vi "strip zeroes.vi"(1 "Array in":dbl[](array[numeric])) -> (0 "Array out":dbl[](array[numeric]))   [LabVIEW 2009]
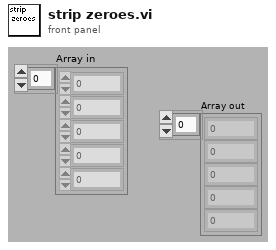
[diagram p1: front panel]
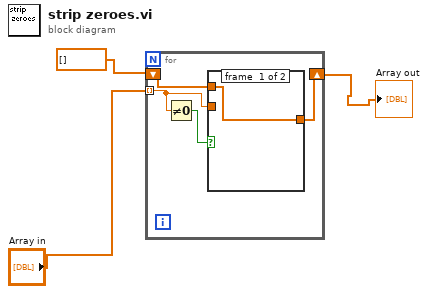
[diagram p0: block diagram]
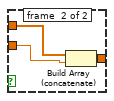
[diagram p2: hidden frame]
diagram:
  n1 = for {
    tunnel: "Array in" -> [w4] mode=indexing
    shift-right: [w6] -> w3
    shift-left: dbl[] [] ("array") -> [w7]
    n2 = Not Equal To 0?(x=w4) -> (x != 0?=w5:bool)
    n3 = case shown="True" w5 {
      tunnel: w7 -> [w8 w11]
      tunnel: [w8 w10] -> w6
      tunnel: w4 -> [_ w9]
      frame #0 {
      }
      frame #1 {
        n4 = Build Array (concatenate)(w11, w9) -> (w10:dbl[])
      }
    }
  }
  "Array out" <- w3
